vi "题目3.vi"() -> ()   [LabVIEW 2017]
panel:
  out "数组":dbl[][](array[numeric])
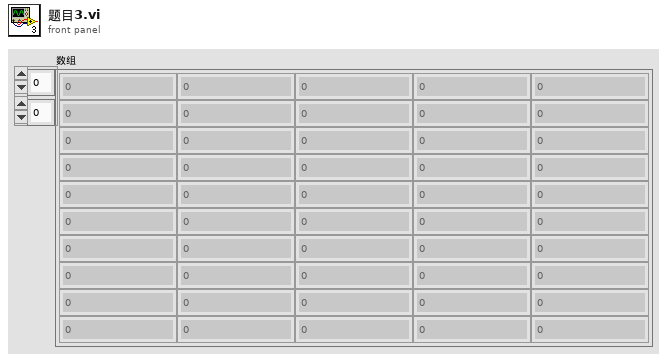
[diagram p1: front panel]
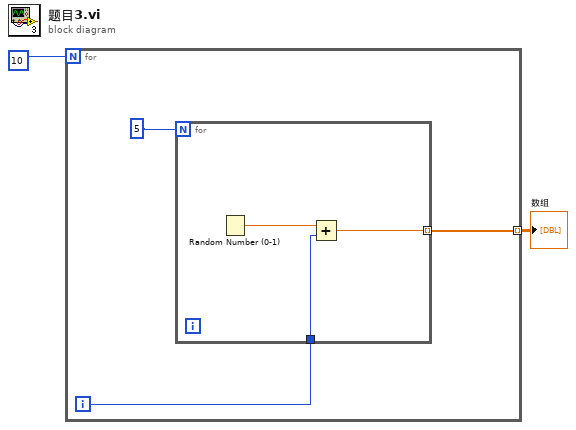
[diagram p0: block diagram]
diagram:
  n1 = for {
    N: 10 -> [_]
    tunnel: [w4] -> w2 mode=indexing
    i -> [w5]
    n2 = for {
      N: 5 -> [_]
      tunnel: w5 -> [w7]
      tunnel: [w6] -> w4 mode=indexing
      n3 = Random Number (0-1)() -> (number: 0 to 1=w8:dbl)
      n4 = Add(x=w8, y=w7) -> (x+y=w6:dbl)
    }
  }
  "数组" <- w2
